vi "Create Scaling.vi"(8 "error in (no error)":errorcluster, 11 "Data Processor Module in":refnum<class "Data Processor Module.lvclass">) -> (0 "error out":errorcluster, 3 "Data Processor Module out":refnum<class "Data Processor Module.lvclass">)   [LabVIEW 2023, in "VolatusData.lvlib" / "Data Processor Module.lvclass"]
uses:
  Data Processor Module.lvclass
  Data Processor Module.lvclass/Data Processor Module.ctl
  VolatusConfig/Meta Type.ctl
  Volatus/Module/Module.lvclass/Module.ctl
  lv-vecto/Vecto/Group/Group.lvclass/Group.ctl
  lv-vecto/Vecto/Group Config/Group Config.lvclass/Group Config.ctl
  VolatusConfig/VolatusConfigElement/VolatusConfigElement.lvclass/VolatusConfigElement.ctl
  VolatusConfig/Group/Group Config.lvclass
  VolatusConfig/VolatusConfigElement/Element.vi
  lv-cdm/CDM-Config/Config Lookup/Match Meta.vi
  lv-cdm/CDM-Config/Config Element/Owner.vi
  lv-cdm/CDM-Config/Config Manager/Lookup Descendant.vi
  VolatusConfig/Scaling/Create (Group).vi
  Scaling/Create (Config).vi
  lv-cdm/CDM-Config/Config Filter/Config Lookup.lvclass
  Volatus/Module/Module.lvclass
  lv-vecto/Vecto/Group/Group.lvclass
  VolatusConfig/VolatusConfig.lvlib
  lv-cdm/CDM-Config/Config Element/Config Element.lvclass
  VolatusConfig/VolatusConfigElement/VolatusConfigElement.lvclass
  Scaling/Scaling.lvclass
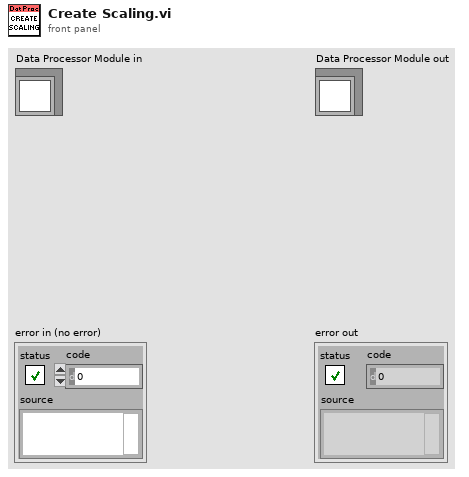
[diagram p1: front panel]
types:
  T1 = typedef "VolatusConfig.lvlib/Meta Type.ctl" = enum16{"UNKNOWN", "VL_System", "VL_Cluster", "VL_Node", "VL_Task", "VL_Group", "VL_Channel", "VL_Task_List", "VL_Scaling", "VL_Sensor", "VL_Sensor_List", "VL_Scale"}
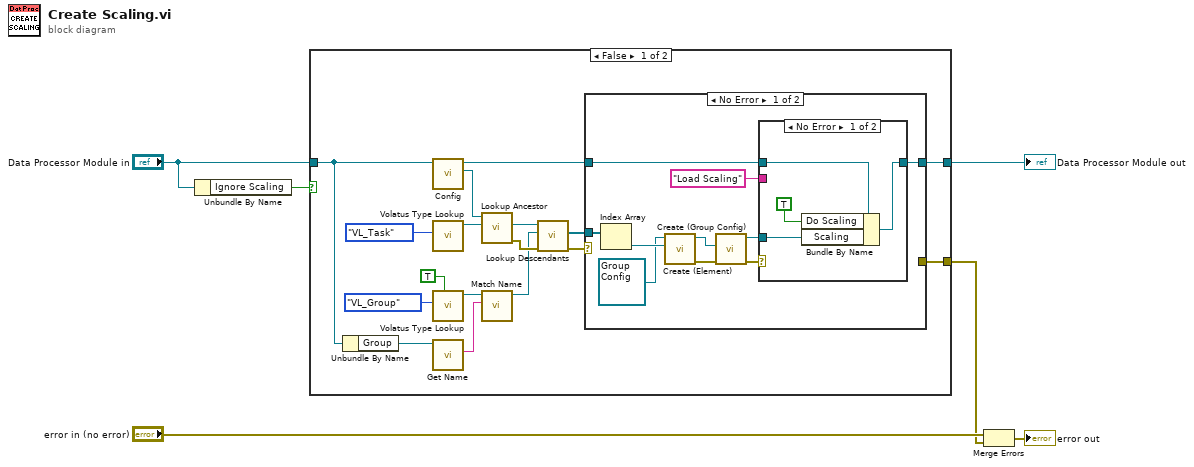
[diagram p0: block diagram]
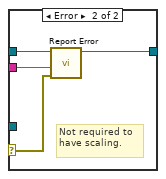
[diagram p2: hidden frame]
diagram:
  n1 = Unbundle By Name("Data Processor Module in") -> ("Ignore Scaling"=w1:bool)
  n2 = case shown="False" w1 {
    tunnel: "Data Processor Module in" -> [w22 w44]
    tunnel: [w9 _] -> w4
    tunnel: [w7 w44] -> w3
    frame False {
      n3 = Unbundle By Name(w22) -> ("Group"=w21:refnum<class "Group.lvclass">)
      n4 = call "Config.vi"("Module in"=w22) -> ("Config"=w20:refnum<class "VolatusConfigElement.lvclass">, "Module out"=w8:refnum<class "Data Processor Module.lvclass">)  [unwired: 9 in]
      n5 = call "Volatus Type Lookup.vi"("Meta Type"=Meta_Type."VL_Task") -> ("Config Lookup out"=w18:refnum<class "Config Lookup.lvclass">)  [unwired: 9 in, 1 out]
      n6 = call "Volatus Type Lookup.vi"("Don't Recurse Past Match (F)"=TRUE, "Meta Type"=Meta_Type."VL_Group") -> ("Config Lookup out"=w15:refnum<class "Config Lookup.lvclass">)  [unwired: 8 in, 1 out]
      n7 = call "Get Name.vi"("Group in"=w21) -> ("Name"=w14:string)  [unwired: 8 in, 2 out]
      n8 = call "Lookup Ancestor.vi"("Lookup"=w18, "VolatusConfigElement in"=w20) -> ("error out"=w23:errorcluster, "Ancestor"=w17:refnum<class "Config Element.lvclass">)  [unwired: 7 in, 1 out]
      n9 = call "Match Name.vi"("Name"=w14, "Config Lookup (New)"=w15) -> ("Config Lookup out"=w13:refnum<class "Config Lookup.lvclass">)  [unwired: 8 in, 1 out]
      n10 = call "Lookup Descendants.vi"("error in (no error)"=w23, "Lookup"=w13, "Config Element in"=w17) -> ("error out"=w10:errorcluster, "Descendants"=w11:refnum<class "Config Element.lvclass">[])  [unwired: 6 in, 1 out]
      n11 = case shown="No Error" w10 {
        selector: w10 -> [_ w43]
        tunnel: w11 -> [w33 _]
        tunnel: [_ w43] -> w9
        tunnel: w8 -> [w27 w42]
        tunnel: [w25 w42] -> w7
        frame No Error {
          n12 = Index Array(array=w33) -> (element=w32:refnum<class "Config Element.lvclass">)  [unwired: 1 in]
          n13 = call "Create (Element).vi"("Element"=w32, "VolatusConfigElement in"=refnum<class "Group Config.lvclass"> refnum ("VolatusConfig.lvlib:Group.lvclass")) -> ("error out"=w29:errorcluster, "VolatusConfigElement out"=w30:refnum<class "Group Config.lvclass">)  [unwired: 8 in]
          n14 = call "Create (Group Config).vi"("error in (no error)"=w29, "Group Config"=w30) -> ("error out"=w28:errorcluster, "Scaling out"=w26:refnum<class "Scaling.lvclass">)  [unwired: 8 in]
          n15 = case shown="No Error" w28 {
            selector: w28 -> [_ w39]
            tunnel: w27 -> [w37 w41]
            tunnel: w26 -> [w36 _]
            tunnel: [w34 w40] -> w25
            tunnel: "Load Scaling" -> [_ w38]
            frame No Error {
              n16 = Bundle By Name(cluster=w37, "Do Scaling"=TRUE, "Scaling"=w36) -> (w34:refnum<class "Data Processor Module.lvclass">)
            }
            frame Error {
              # "Not required to have scaling."
              n17 = call "Report Error.vi"("error in (no error)"=w39, "Message (None)"=w38, "Module in"=w41) -> ("Module out"=w40:refnum<class "Data Processor Module.lvclass">)  [unwired: 7 in, 1 out]
            }
          }
        }
        frame Error {
        }
      }
    }
    frame True {
      # "Scaling turned off even though channels might have scaling configuration. This is likely the case with output modules (DAQmxAO, DAQmxDO) that have already scaled values directly."
    }
  }
  "Data Processor Module out" <- w3
  n18 = Merge Errors("error in (no error)", w4) -> (→"error out":errorcluster)
